vi "Performance Values.vi"(8 "error in (no error)":errorcluster, 11 "Windows System SAL in":refnum<class "Windows System SAL.lvclass">) -> (0 "error out":errorcluster, 2 "Performance Values":T1)   [LabVIEW 2020, in "Volatus.lvlib" / "Windows System SAL.lvclass"]
uses:
  Windows System SAL.lvclass
  System SAL/Performance Values.ctl
  Windows System SAL.lvclass/Windows System SAL.ctl
  System SAL/System SAL.lvclass
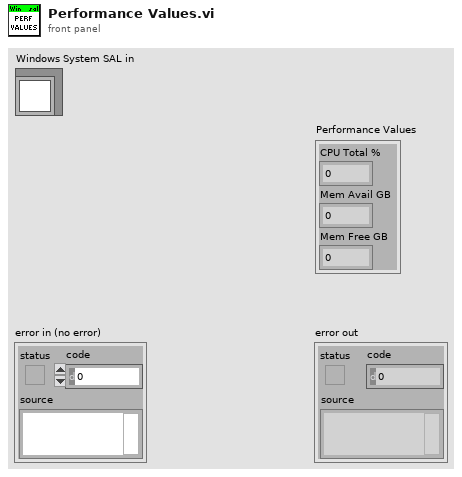
[diagram p1: front panel]
types:
  T1 = typedef "Volatus.lvlib/System SAL.lvclass/Performance Values.ctl" = cluster{"CPU Total %":dbl, "Mem Avail GB":dbl, "Mem Free GB":dbl}
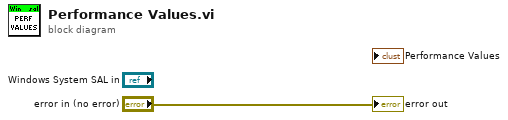
[diagram p0: block diagram]
diagram:
  "error out" <- "error in (no error)"
